vi "sub_waypoint_update_all.vi"(11 "waypoint files cfg":T1={"Waypoint array"=[{"sel"=TRUE, "inv"=FALSE, "path"=path "C:/AGV/Log/0709/refwpt_0709-1 parking-lot to cafe.txt"}, {"sel"=TRUE, "inv"=TRUE, "path"=path "C:/AGV/Log/0709/refwpt_0709-3 hill to cafe.txt"}, {"sel"=TRUE, "inv"=FALSE, "path"=path "C:/AGV/Log/0709/refwpt_0709-3 hill to cafe.txt"}, {"sel"=TRUE, "inv"=TRUE, "path"=path "C:/AGV/Log/0709/refwpt_0709-1 parking-lot to cafe.txt"}]}) -> (3 "Total map cfg":T2(graph))   [LabVIEW 2019]
uses:
  Ctrl/waypoint_buf.ctl
  Ctrl/cmd_ini-RW.ctl
panel:
  out "wpt count":i32
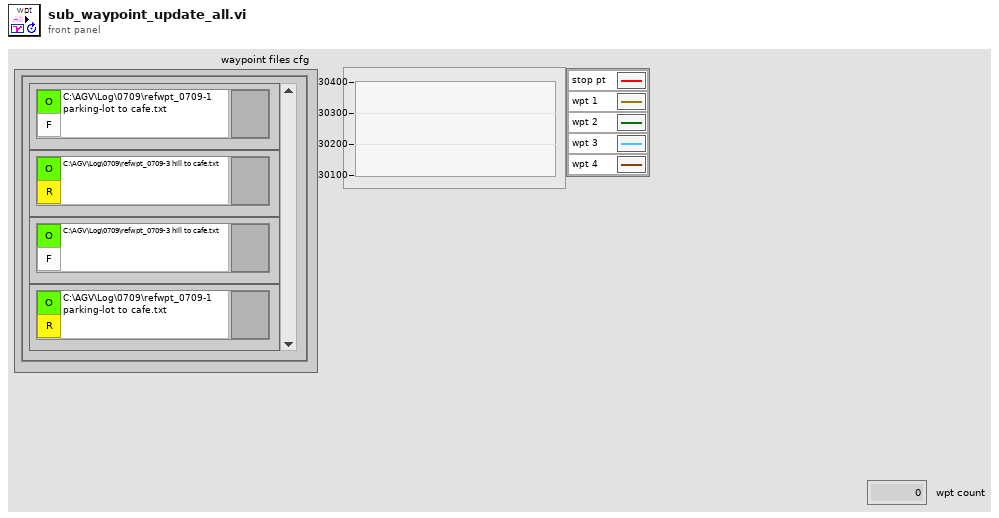
[diagram p1: front panel]
types:
  T1 = cluster{"Waypoint array":cluster{"sel":bool, "inv":bool, "path":path}[]}
  T2 = cluster{"ref waypt 0703 A \ngoal point start":cluster{"X":dbl, "Y":dbl}[]}[]
  T3 = typedef "cmd_ini-RW.ctl" = enum16{"ini", "read", "write"}
  T4 = typedef "waypoint_buf.ctl" = enum16{"clear", "write", "read"}
  T5 = cluster{"wpt group i":i32, "state total i":i32, "state main i":i32}
  T6 = typedef "status.ctl" = u16
  T7 = cluster{"AGV":T6, "AGV Estop":T6, "Obstacle":T6, "Heading":T6, "Waypt":T6, "GNSS":T6, "VLP16":T6, "Cam":T6, "RPLidar":T6, "Joystick":T6}
  T8 = typedef "statistics_val.ctl" = cluster{"gap plus mean":dbl, "gap plus max":dbl, "gap plus sum":dbl, "gap minus mean":dbl, "gap minus max":dbl, "gap minus sum":dbl, "gap abs mean":dbl, "gap abs max":dbl, "gap abs sum":dbl, "wpt length":dbl, "total moving time":dbl, "average speed":dbl, "plus gap count":u64, "minus gap count":u64, "drive length":dbl}
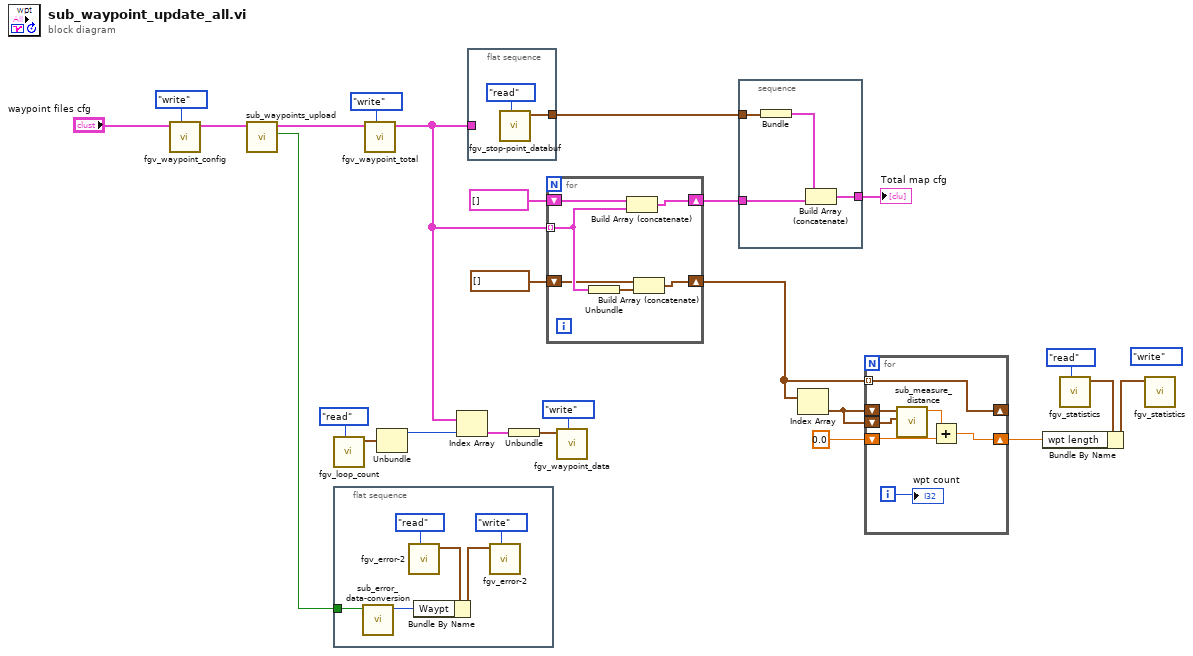
[diagram p0: block diagram]
diagram:
  (unwired) cmd_ini-RW."write" ("cmd")
  n1 = call "fgv_waypoint_config.vi"("cmd"=enum16{"read", "write"}."write", "waypoint files cfg"="waypoint files cfg") -> ("waypoint files cfg out"=w10:T1)  [unwired: 9 in]
  n2 = call "sub_waypoints_upload.vi"("waypoint group"=w10) -> ("waypt error"=w14:bool, "waypoint all"=w21:cluster{"XY 그래프":cluster{"X":dbl, "Y":dbl}[]}[])  [unwired: 9 in]
  n3 = call "fgv_loop_count.vi"("cmd"=enum16{"init", "read", "write"}."read") -> ("loop count out"=w18:T5)  [unwired: 9 in, 1 out]
  n4 = flat-sequence {
    tunnel: w14 -> [w26]
    frame #0 {
      n5 = call "sub_error_data-conversion.vi"("error status"=w26) -> ("error conversion out"=w27:T6)  [unwired: 9 in, 1 out]
      n6 = call "fgv_error-2.vi"("cmd"=enum16{"init", "read", "write"}."read") -> ("Error cluster out"=w30:T7)  [unwired: 9 in, 1 out]
      n7 = Bundle By Name(cluster=w30, "Waypt"=w27) -> (w31:T7)
      n8 = call "fgv_error-2.vi"("cmd"=enum16{"init", "read", "write"}."write", "Error cluster"=w31) -> ()  [unwired: 8 in, 2 out]
    }
  }
  n9 = call "fgv_waypoint_total.vi"("cmd"=enum16{"write", "read"}."write", "waypoint total in"=w21) -> ("waypoint total out"=w13:cluster{"waypt":cluster{"X":dbl, "Y":dbl}[]}[])  [unwired: 9 in]
  n10 = Unbundle(w18) -> ("wpt group i"=w17:i32)  [unwired: 2 out]
  n11 = Index Array(array=w13, index=w17) -> (element=w16:cluster{"waypt":cluster{"X":dbl, "Y":dbl}[]})
  n12 = flat-sequence {
    tunnel: [w32] -> w22
    tunnel: w13 -> [_]
    frame #0 {
      n13 = call "fgv_stop-point_databuf.vi"("cmd"=enum16{"clear", "write", "read"}."read") -> ("all stop pts out"=w32:cluster{dbl, dbl}[])  [unwired: 10 in]
    }
  }
  n14 = Unbundle(w16) -> ("waypt"=w15:cluster{"X":dbl, "Y":dbl}[])
  n15 = for {
    shift-right: [w38] -> w8
    shift-left: T2 [] -> [w39]
    tunnel: w13 -> [w37] mode=indexing
    shift-right: [w36] -> w1
    shift-left: cluster{"X":dbl, "Y":dbl}[] [] -> [w35]
    n16 = Unbundle(w37) -> ("waypt"=w34:cluster{"X":dbl, "Y":dbl}[])
    n17 = Build Array (concatenate)(w39, w37) -> (w38:cluster{"waypt":cluster{"X":dbl, "Y":dbl}[]}[])
    n18 = Build Array (concatenate)(w35, w34) -> (w36:cluster{"X":dbl, "Y":dbl}[])
  }
  n19 = call "fgv_waypoint_data.vi"("cmd"=waypoint_buf."write", "waypoint in"=w15) -> ()  [unwired: 7 in, 3 out]
  n20 = stacked-sequence {
    tunnel: [w42] -> w23
    tunnel: w8 -> [w43]
    tunnel: w22 -> [w41]
    frame #0 {
      n21 = Bundle("all stop pts out"=w41) -> (w40:cluster{"all stop pts out":cluster{dbl, dbl}[]})  [unwired: 1 in]
      n22 = Build Array (concatenate)(w40, w43) -> (w42:T2)
    }
  }
  "Total map cfg" <- w23
  n23 = Index Array(array=w1) -> (element=w3:cluster{"X":dbl, "Y":dbl})  [unwired: 1 in]
  n24 = for {
    tunnel: w1 -> [w50] mode=indexing
    shift-right: [w50] -> _
    shift-left: w3 -> [w49]
    shift-left: w3 -> [w48]
    shift-right: [w45] -> w2
    shift-left: 0.0 -> [w47]
    i -> [w44]
    n25 = call "sub_measure_distance.vi"("pt 2"=w48, "pt 1"=w49) -> ("distance"=w46:dbl)  [unwired: 9 in]
    n26 = Add(x=w46, y=w47) -> (x+y=w45:dbl)
    "wpt count" <- w44
  }
  n27 = call "fgv_statistics.vi"("cmd"=cmd_ini-RW."read") -> ("statistics values out"=w7:T8)  [unwired: 10 in]
  n28 = Bundle By Name(cluster=w7, "wpt length"=w2) -> (w6:T8)
  n29 = call "fgv_statistics.vi"("statistics values"=w6) -> ()  [unwired: 10 in, 1 out]
